vi "VL Type.vi"(8 "error in (no error)":errorcluster, 11 "Scaling in":refnum<class "Scaling.lvclass">) -> (0 "error out":errorcluster, 2 "VL Type":T1, 3 "Scaling out":refnum<class "Scaling.lvclass">)   [LabVIEW 2020, in "VolatusConfig.lvlib" / "Scaling.lvclass"]
uses:
  Scaling.lvclass
  Meta Type.ctl
  Scaling.lvclass/Scaling.ctl
  VolatusConfig.lvlib
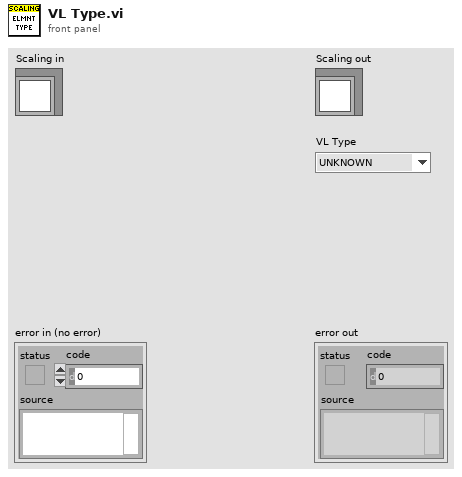
[diagram p1: front panel]
types:
  T1 = typedef "VolatusConfig.lvlib/Meta Type.ctl" = enum16{"UNKNOWN", "VL_System", "VL_Cluster", "VL_Node", "VL_Task", "VL_Group", "VL_Channel", "VL_Task_List", "VL_Scaling"}
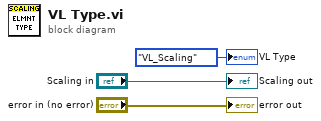
[diagram p0: block diagram]
diagram:
  "error out" <- "error in (no error)"
  "Scaling out" <- "Scaling in"
  "VL Type" <- Meta_Type."VL_Scaling" ("VL Type")
